vi "Laser Controller.vi"() -> ()   [LabVIEW 2022 SP3]
uses:
  <vilib>/MakerHub/LINX/Public/Utilities/Open Serial.vi
  <vilib>/MakerHub/LINX/LMH-LINX.lvlib
panel:
  in  "Trigger Pin":u8
  in  "Laser Pin":u8
  in  "milliseconds to wait":u32
  in  "Stop Button":bool
  in  "Serial Port":refnum<visa-resource-name>="N/A"
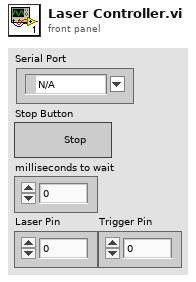
[diagram p1: front panel]
types:
  T1 = typedef "LMH-LINX.lvlib/LINX Ref.ctl" = cluster{"IO":T2, "Interface":T3, "LINX Device Config":T4}
  T2 = typedef "LMH-LINX.lvlib/Platform.ctl" = enum16{"Remote", "Local"}
  T3 = typedef "LMH-LINX.lvlib/Interface.ctl" = enum16{"Serial", "TCP"}
  T4 = typedef "LMH-LINX.lvlib/Device.lvlib/LINX Device Config.ctl" = cluster{"Interface":T3, "COM Port":refnum<visa-resource-name>, "TCP Configuration":T5, "Device Family":u8, "Device ID":u8, "Device Name":string, "TCP Ref":refnum<k5>, "Channels":T6}
  T5 = typedef "LMH-LINX.lvlib/Device.lvlib/TCP Config.ctl" = cluster{"IP Address":string, "Port":u16}
  T6 = typedef "LMH-LINX.lvlib/Channels.ctl" = cluster{"DI":u8[], "DO":u8[], "AI":u8[], "AO":u8[], "PWM":u8[], "QE":u8[], "UART":u8[], "I2C 2":u8[], "SPI":u8[], "CAN":u8[], "Servo":u8[], "AI Ref (V)":dbl, "AI Resolution (Bits)":u8, "AO Ref (V)":dbl, "AO Resolution (Bits)":u8}
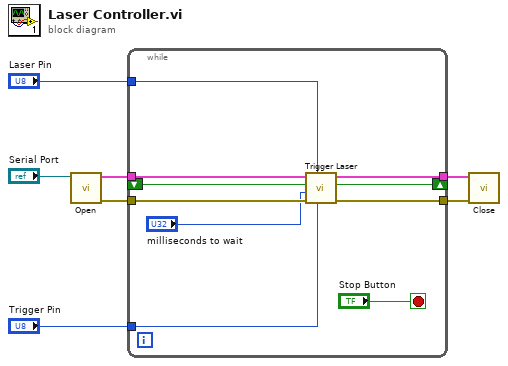
[diagram p0: block diagram]
diagram:
  n1 = call-poly <vilib>:"Open.vi"("Serial Port"="Serial Port") -> ("Error Out"=w5:errorcluster, "LINX Resource"=w7:T1)  [unwired: 8 in, 1 out]
  n2 = while {
    tunnel: w7 -> [w17]
    tunnel: [w16] -> w6
    tunnel: w5 -> [w15]
    tunnel: [w8] -> w4
    shift-right: [w14] -> _
    shift-left: _ -> [w13]
    tunnel: "Laser Pin" -> [w12]
    tunnel: "Trigger Pin" -> [w10]
    stop <- "Stop Button" stop-if-true
    n3 = call "Trigger Laser.vi"("Trigger Pin"=w10, "Laser Pin"=w12, "error in (no error)"=w15, "milliseconds to wait"="milliseconds to wait", "DI Value in"=w13, "LINX Resource in"=w17) -> ("error out"=w8:errorcluster, "DI Value out"=w14:bool, "LINX Resource out"=w16:T1)  [unwired: 1 in]
  }
  n4 = call <vilib>:"Close.vi"("Error In"=w4, "LINX Resource"=w6) -> ()  [unwired: 9 in, 1 out]
